vi "Callback.vi"(4 "User Event":refnum<user-event>, 5 "Event Data":cluster{"sender":refnum<k24>, "e":refnum<k24>}, 6 "Control Ref":refnum<k24>, 7 "Event Common Data":T1) -> ()   [LabVIEW 2017]
uses:
  System.Windows.Forms
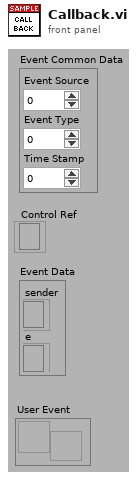
[diagram p1: front panel]
types:
  T1 = cluster{"Event Source":i32, "Event Type":u32, "Time Stamp":u32}
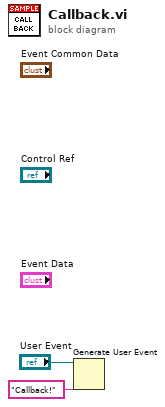
[diagram p0: block diagram]
diagram:
  n1 = Generate User Event(user event="User Event", event data cluster="Callback!" ("event data")) -> ()  [unwired: 2 in, 2 out]
